vi "acquire_digital_inputs.vi"(5 "Error In":errorcluster) -> (19 "Error Out":errorcluster)   [LabVIEW 2013, in "examples.lvlib"]
doc: "Demonstrates the ability to read the status of the referenced controller's digital inputs. Refer to the front panel for instructions.\n\nProduced By:\n\n<B>Kod Integrations, LLC</B>\n4835 Marianne Drive\nMount Airy, MD 21771\nhttp://www.kodintegrations.com\nemail: info@kodintegrations.com\nphone: (240) 687-1288"
uses:
  libraries/examples.lvlib
  classes/Controller/_Controller.lvclass
  common/controls/digital_input.ctl
  libraries/common.lvlib
  common/controls/digital_input_item.ctl
panel:
  out "di_items":T1[](array[typedef])
  out "dig_val (single only)":bool
  in  "get_all? (def=F)":bool
  in  "di (single)":T2
  in  "clear_buffer? (T)":bool=TRUE
  in  "device_index (in) [0=def]":i32
  # "instructions:\n\nThis VI can retrieve the status of ALL digital\ninputs or just a single one.  If retrieving ALL, \nset the input \"get_all?\" to TRUE and run the VI.\n\nIf retrieve just one, set the in put \"get_all?\" to\nFALSE (the default value) and select the digital\ninput value with the \"di (single)\" input."
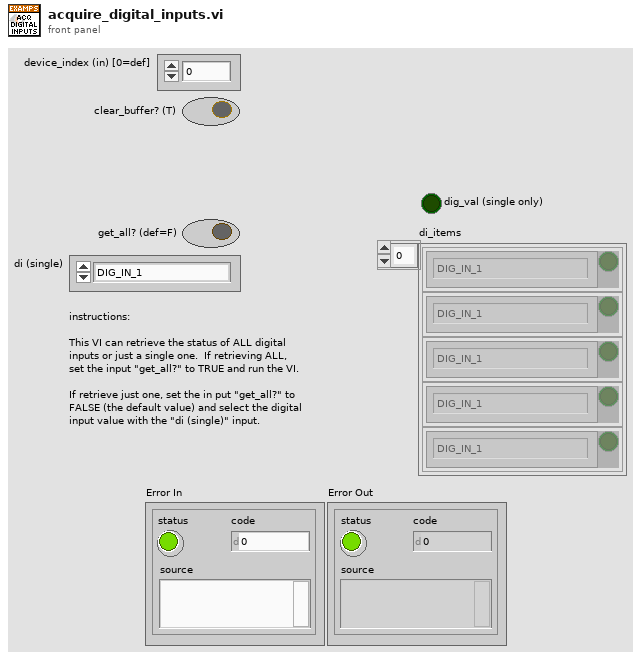
[diagram p1: front panel]
types:
  T1 = typedef "common.lvlib/digital_input_item.ctl" = cluster{"item":T2, "status":bool}
  T2 = typedef "common.lvlib/digital_input.ctl" = enum16{"DIG_IN_1", "DIG_IN_2", "DIG_IN_3", "DIG_IN_4", "DIG_IN_5", "DIG_IN_6", "DIG_IN_7", "DIG_IN_8", "NEG_LIMIT", "HOME", "POS_LIMIT"}
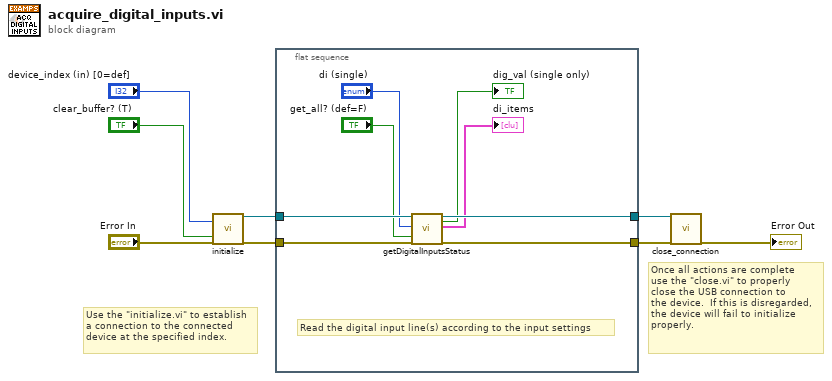
[diagram p0: block diagram]
diagram:
  # "Once all actions are complete\nuse the \"close.vi\" to properly\nclose the USB connection to \nthe device.  If this is disregarded,\nthe device will fail to initialize \nproperly."
  # "Use the \"initialize.vi\" to establish\na connection to the connected\ndevice at the specified index."
  n1 = call "initialize.vi"("device_index (in) [0=def]"="device_index (in) [0=def]", "clear_buffer? (T)"="clear_buffer? (T)", "error in (no error)"="Error In") -> ("reference (out)"=w5:refnum<class "_Controller.lvclass">, "error out"=w4:errorcluster)  [unwired: 15 in]
  n2 = flat-sequence {
    tunnel: w5 -> [w16]
    tunnel: w4 -> [w15]
    tunnel: [w14] -> w3
    tunnel: [w13] -> w2
    frame #0 {
      # "Read the digital input line(s) according to the input settings"
      n3 = call "getDigitalInputsStatus.vi"("Controller in"=w16, "di (single)"="di (single)", "get_all? (def=F)"="get_all? (def=F)", "error in (no error)"=w15) -> ("Controller out"=w14:refnum<class "_Controller.lvclass">, "dig_val (single only)"=→"dig_val (single only)":bool, "di_items"=→"di_items":T1[], "error out"=w13:errorcluster)  [unwired: 11 in, 1 out]
    }
  }
  n4 = call "close_connection.vi"("reference (in)"=w3, "error in (no error)"=w2) -> ("error out"=→"Error Out":errorcluster)  [unwired: 16 in, 1 out]
